vi "LaserSync_VI.vi"() -> ()   [LabVIEW 2015]
uses:
  <vilib>/Platform/TimedLoop/XDataNode/timing_clust.ctl
  <vilib>/Platform/TimedLoop/XDataNode/nitl_modes.ctl
  <vilib>/Platform/TimedLoop/XDataNode/wakeup.ctl
  <vilib>/FPGAPlugInAG/myRIO-1950/niLvFpga_Open_myRIO-1950.vi
  <vilib>/rvi/interface/common/dynamic/niFpgaDynamicAddResources.vi
  <vilib>/Utility/error.llb/Error Cluster From Error Code.vi
  <vilib>/rvi/errors/niLvFpgaAdjustHostInterfaceError.vi
  <vilib>/RVI Host/nirviSupport.llb/nirviErrorClusterFromErrorCode.vi
  <vilib>/Analysis/3filter.llb/Butterworth Filter (DBL).vi
  <vilib>/FPGAPlugInAG/Dynamic/niLvFpga_Close_Dynamic.vi
  <vilib>/Analysis/Matrix/Numeric/Conversions/Array To Matrix - RA.vi
  <vilib>/Platform/TimedLoop/XDataNode/XDataNode.xnode
  <vilib>/rvi/interface/nirviOpenFPGA/nirviOpenFPGA.xnode
  FPGA Bitfiles/Flylaserbox_FPGATarget_FPGAsingleloop_H8b3XToqd60.lvbitx
  FPGA_single_loop.vi
  <vilib>/rvi/interface/nirviReadWriteControl/nirviReadWriteControl.xnode
  <vilib>/rvi/interface/nirviMethod/nirviMethod.xnode
  <vilib>/rvi/interface/nirviCloseFPGA/nirviCloseFPGA.xnode
  <vilib>/Platform/TimedLoop/XDataNode/XDNodeRunTimeDep.lvlib
  <vilib>/rvi/interface/Simulation/niFpgaSimulationCallBeginRW.vi
  <vilib>/rvi/interface/nirviMethod/StockFPGA_InlinedMethodWaitForSingleIRQ.vi
  <vilib>/FPGAPlugInAG/Dynamic/niLvFpga_WaitOnIrq_Dynamic.vi
  <vilib>/FPGAPlugInAG/Dynamic/niLvFpga_ReadFifo_Dynamic.vi
  <vilib>/rvi/errors/niLvFpgaMergeErrorWithErrorCode.vi
  <vilib>/FPGAPlugInAG/Dynamic/niLvFpga_AcknowledgeIrq_Dynamic.vi
  <vilib>/Analysis/NI_AALBase.lvlib
  <vilib>/Analysis/Matrix/NI_Matrix.lvlib
  NiFpgaLv.dll
panel:
  in  "Laser On? All lasers":bool
  in  "Laser J8":u16=2855
  in  "Laser J5":u16=749
  in  "Laser J4":u16=766
  in  "Laser J1":u16=3000
  out "Loop count of LED":i32=6674
  in  "Producer Loop Stop-2":bool
  in  "Producer Loop Stop":bool
  out "Consumer Loop Time":u32=20
  out "Host VI loop count":i32=33366
  out "Noise check":dbl[](graph)
  out "Fly real-time location":dbl(graph)=245.7942691305756
  in  "Choose which setup to look at":dbl=2.0
  out "Display Raw Data":dbl[](graph)=[329.0, 351.0, 375.0, 381.0, 409.0, 416.0, 442.0, 448.0, 474.0, 481.0, 503.0, 511.0, 538.0, 543.0, 569.0, 571.0, 596.0, 603.0, 622.0, 627.0, 644.0, 647.0, 671.0, 666.0, 687.0, 687.0, 703.0, 701.0, 719.0, 713.0, 728.0, 726.0, 740.0, 733.0, 743.0, 736.0, 749.0, 742.0, 754.0, 743.0, 751.0, 742.0, 752.0, 741.0, 755.0, 747.0, 758.0, 752.0, 763.0, 754.0, 764.0, 757.0, 772.0, 762.0, 774.0, 766.0, 779.0, 769.0, 780.0, 770.0, 782.0, 770.0, 779.0, 769.0, 781.0, 773.0, 788.0, 777.0, 788.0, 780.0, 794.0, 785.0, 799.0, 792.0, 806.0, 801.0, 813.0, 808.0, 821.0, 814.0, 828.0, 821.0, 833.0, 826.0, 838.0, 830.0, 842.0, 830.0, 840.0, 834.0, 848.0, 838.0, 849.0, 837.0, 849.0, 840.0, 854.0, 842.0, 853.0, 848.0, 861.0, 849.0, 860.0, 854.0, 868.0, 855.0, 867.0, 859.0, 872.0, 863.0, 873.0, 865.0, 881.0, 871.0, 883.0, 874.0, 883.0, 877.0, 889.0, 880.0, 892.0, 879.0, 895.0, 887.0, 897.0, 885.0, 891.0, 881.0, 883.0, 894.0, 900.0, 897.0, 908.0, 907.0, 915.0, 912.0, 923.0, 921.0, 927.0, 926.0, 936.0, 934.0, 938.0, 937.0, 943.0, 936.0, 945.0, 941.0, 949.0, 943.0, 954.0, 951.0, 963.0, 960.0, 969.0, 968.0, 977.0, 974.0, 983.0, 981.0, 989.0, 986.0, 998.0, 991.0, 999.0, 995.0, 1002.0, 1002.0, 1004.0, 1002.0, 1006.0, 1002.0, 1014.0, 1007.0, 1016.0, 1013.0, 1020.0, 1013.0, 1022.0, 1015.0, 1019.0, 1016.0, 1021.0, 1018.0, 1022.0, 1015.0, 1021.0, 1012.0, 1019.0, 1013.0, 1015.0, 1014.0, 1018.0, 1009.0, 1019.0, 1014.0, 1019.0, 1015.0, 1020.0, 1016.0, 1024.0, 1012.0, 1020.0, 1013.0, 1017.0, 1015.0, 1025.0, 1020.0, 1029.0, 1021.0, 1027.0, 1023.0, 1028.0, 1018.0, 1025.0, 1021.0, 1026.0, 1017.0, 1019.0, 1013.0, 1016.0, 1004.0, 1007.0, 1006.0, 1007.0, 1000.0, 1001.0, 989.0, 994.0, 985.0, 989.0, 986.0, 988.0, 983.0, 987.0, 979.0, 983.0, 978.0, 984.0, 976.0, 984.0, 975.0, 983.0, 978.0, 983.0, 978.0, 986.0, 981.0, 984.0, 970.0, 978.0, 975.0, 981.0, 973.0, 968.0, 951.0, 999.0, 1012.0, 1013.0, 1012.0, 1009.0, 1010.0, 1012.0, 1017.0, 1016.0, 1019.0, 1021.0, 1028.0, 1030.0, 1035.0, 1037.0, 1043.0, 1047.0, 1052.0, 1054.0, 1061.0, 1064.0, 1069.0, 1074.0, 1080.0, 1082.0, 1087.0, 1089.0, 1091.0, 1095.0, 1099.0, 1096.0, 1098.0, 1099.0, 1103.0, 1106.0, 1110.0, 1112.0, 1115.0, 1119.0, 1124.0, 1123.0, 1127.0, 1127.0, 1130.0, 1132.0, 1134.0, 1134.0, 1137.0, 1134.0, 1137.0, 1139.0, 1139.0, 1139.0, 1139.0, 1138.0, 1142.0, 1141.0, 1139.0, 1139.0, 1139.0, 1135.0, 1135.0, 1133.0, 1138.0, 1137.0, 1137.0, 1136.0, 1135.0, 1131.0, 1133.0, 1131.0, 1132.0, 1129.0, 1129.0, 1127.0, 1126.0, 1119.0, 1120.0, 1120.0, 1119.0, 1115.0, 1114.0, 1111.0, 1109.0, 1107.0, 1106.0, 1104.0, 1102.0, 1102.0, 1102.0, 1101.0, 1098.0, 1097.0, 1097.0, 1095.0, 1103.0, 1095.0, 1097.0, 1095.0, 1099.0, 1099.0, 1101.0, 1099.0, 1105.0, 1104.0, 1105.0, 1110.0, 1112.0, 1112.0, 1114.0, 1116.0, 1114.0, 1114.0, 1113.0, 1116.0, 1118.0, 1117.0, 1119.0, 1117.0, 1121.0, 1122.0, 1123.0, 1123.0, 1125.0, 1122.0, 1127.0, 1130.0, 1127.0, 1118.0, 1129.0, 1126.0, 1125.0, 1114.0, 1114.0, 1107.0, 1109.0, 1101.0, 1105.0, 1101.0, 1103.0, 1097.0, 1103.0, 1097.0, 1105.0, 1098.0, 1099.0, 1096.0, 1101.0, 1099.0, 1103.0, 1101.0, 1105.0, 1099.0, 1104.0, 1101.0, 1106.0, 1098.0, 1101.0, 1096.0, 1098.0, 1091.0, 1096.0, 1093.0, 1097.0, 1094.0, 1098.0, 1093.0, 1099.0, 1093.0, 1099.0, 1096.0, 1102.0, 1102.0, 1108.0, 1107.0, 1113.0, 1110.0, 1114.0, 1114.0, 1120.0, 1116.0, 1122.0, 1120.0, 1128.0, 1125.0, 1131.0, 1130.0, 1136.0, 1131.0, 1135.0, 1133.0, 1140.0, 1137.0, 1143.0, 1139.0, 1141.0, 1138.0, 1139.0, 1137.0, 1145.0, 1142.0, 1144.0, 1138.0, 1149.0, 1148.0, 1153.0, 1147.0, 1150.0, 1145.0, 1149.0, 1144.0, 1147.0, 1140.0, 1144.0, 1139.0, 1144.0, 1137.0, 1142.0, 1139.0, 1144.0, 1139.0, 1142.0, 1137.0, 1142.0, 1138.0, 1144.0, 1141.0, 1144.0, 1143.0, 1150.0, 1147.0, 1156.0, 1154.0, 1157.0, 1157.0, 1161.0, 1157.0, 1162.0, 1160.0, 1166.0, 1160.0, 1168.0, 1163.0, 1171.0, 1166.0, 1170.0, 1165.0, 1171.0, 1167.0, 1170.0, 1165.0, 1169.0, 1165.0, 1172.0, 1170.0, 1185.0, 1094.0, 1101.0, 1108.0, 1099.0, 1106.0, 1104.0, 1101.0, 1100.0, 1103.0, 1099.0, 1099.0, 1094.0, 1098.0, 1089.0, 1093.0, 1086.0, 1088.0, 1081.0, 1083.0, 1078.0, 1082.0, 1074.0, 1074.0, 1069.0, 1073.0, 1066.0, 1065.0, 1060.0, 1065.0, 1058.0, 1060.0, 1055.0, 1053.0, 1053.0, 1053.0, 1047.0, 1048.0, 1043.0, 1051.0, 1045.0, 1047.0, 1042.0, 1045.0, 1038.0, 1043.0, 1038.0, 1040.0, 1038.0, 1044.0, 1041.0, 1043.0, 1037.0, 1042.0, 1037.0, 1036.0, 1035.0, 1040.0, 1033.0, 1039.0, 1033.0, 1036.0, 1035.0, 1036.0, 1032.0, 1032.0, 1032.0, 1035.0, 1028.0, 1036.0, 1034.0, 1037.0, 1032.0, 1034.0, 1031.0, 1033.0, 1030.0, 1034.0, 1026.0, 1028.0, 1026.0, 1030.0, 1022.0, 1028.0, 1021.0, 1023.0, 1020.0, 1019.0, 1014.0, 1012.0, 1009.0, 1010.0, 1004.0, 1008.0, 1002.0, 1003.0, 995.0, 997.0, 987.0, 991.0, 989.0, 987.0, 978.0, 978.0, 974.0, 978.0, 970.0, 973.0, 964.0, 964.0, 958.0, 961.0, 956.0, 954.0, 948.0, 950.0, 946.0, 945.0, 939.0, 938.0, 934.0, 935.0, 930.0, 928.0, 921.0, 923.0, 911.0, 905.0, 898.0, 899.0, 917.0, 903.0, 915.0, 901.0, 913.0, 899.0, 914.0, 897.0, 908.0, 894.0, 906.0, 889.0, 903.0, 887.0, 900.0, 884.0, 899.0, 880.0, 892.0, 877.0, 886.0, 875.0, 887.0, 870.0, 883.0, 868.0, 878.0, 862.0, 875.0, 861.0, 873.0, 857.0, 867.0, 850.0, 864.0, 848.0, 859.0, 844.0, 853.0, 837.0, 847.0, 829.0, 840.0, 822.0, 829.0, 810.0, 822.0, 805.0, 814.0, 802.0, 814.0, 801.0, 814.0, 799.0, 811.0, 797.0, 809.0, 793.0, 803.0, 790.0, 798.0, 788.0, 798.0, 783.0, 794.0, 780.0, 787.0, 776.0, 788.0, 772.0, 781.0, 772.0, 780.0, 767.0, 780.0, 768.0, 771.0, 760.0, 770.0, 751.0, 763.0, 749.0, 761.0, 743.0, 741.0, 709.0, 722.0, 730.0, 737.0, 728.0, 737.0, 724.0, 732.0, 719.0, 723.0, 712.0, 717.0, 701.0, 704.0, 690.0, 695.0, 678.0, 682.0, 664.0, 666.0, 647.0, 645.0, 623.0, 626.0, 606.0, 603.0, 581.0, 576.0, 554.0, 551.0, 529.0, 520.0, 499.0, 490.0, 471.0, 462.0, 443.0, 433.0, 414.0, 405.0, 381.0, 374.0, 268.0, 323.0]
  in  "Fly presence? J8":bool=TRUE
  in  "Threshhold position filter J8":i32=25
  in  "Fly presence? J5":bool=TRUE
  in  "Threshhold position filter J5":i32=25
  in  "Fly presence? J4":bool=TRUE
  in  "Threshhold position filter J4":i32=25
  in  "Threshhold position filter J1":i32=25
  in  "Fly presence? J1":bool=TRUE
  in  "Threshold for noise filter J4":dbl=7.0
  in  "Threshold for noise filter J5":dbl=6.0
  in  "Threshold for noise filter J8":dbl=8.0
  in  "Threshold for noise filter J1":dbl=8.0
  in  "Consumer Loop Stop":bool
  out "Has timed loop ever been late?":bool
  out "Finished Late? [i-1]":bool
  in  "Sensor loop time":i64=20
  in  "Gender J4":string="M"
  in  "Date":string="2017June25"
  in  "Testname J4":string="A"
  in  "Gender J8":string="M"
  in  "Date":string="2017June25"
  in  "Fly J8":i32=4
  in  "Testname Code J8":string="A"
  in  "Fly J4":i32=2
  in  "Gender J5":string="M"
  in  "Date":string="2017June25"
  in  "Fly J5":i32=3
  in  "Testname Code J5":string="A"
  in  "Gender J1":string="F"
  in  "Date":string="2017June25"
  in  "Fly J1":i32=1
  in  "Testname J1":string="A"
  in  "FPGA Stop":bool
  in  "LED switch-2 J8":bool=TRUE
  in  "LED switch-1 J8":bool=TRUE
  in  "LED switch-2 J5":bool=TRUE
  in  "LED switch-1 J5":bool=TRUE
  in  "LED switch-2 J4":bool=TRUE
  in  "LED switch-1 J4":bool=TRUE
  in  "LED switch-2 J1":bool=TRUE
  in  "LED switch-1 J1":bool=TRUE
  in  "LED intensity J8":u32=1000
  in  "LED intensity J5":u32=1000
  in  "LED intensity J4":u32=2500
  in  "LED intensity J1":u32=1000
  out "Frame Count":i16=6056
  out "Host loop time":u32=13
  in  "FIFO Timeout setting (ms)":i32=5000
  out "Elements Remaining Real":u32
  out "Elements Remaining":u32=3080
  out "IRQ(s) Asserted":i32
  out "Sensor Loop Time (FPGA)":u32=11
  out "LED loop time":u32=4000
  out "Iteration Duration":dbl=4.0 format="%#_6f"
  # "0: None\n1: J1\n2: J4\n3: J5\n4: J8"
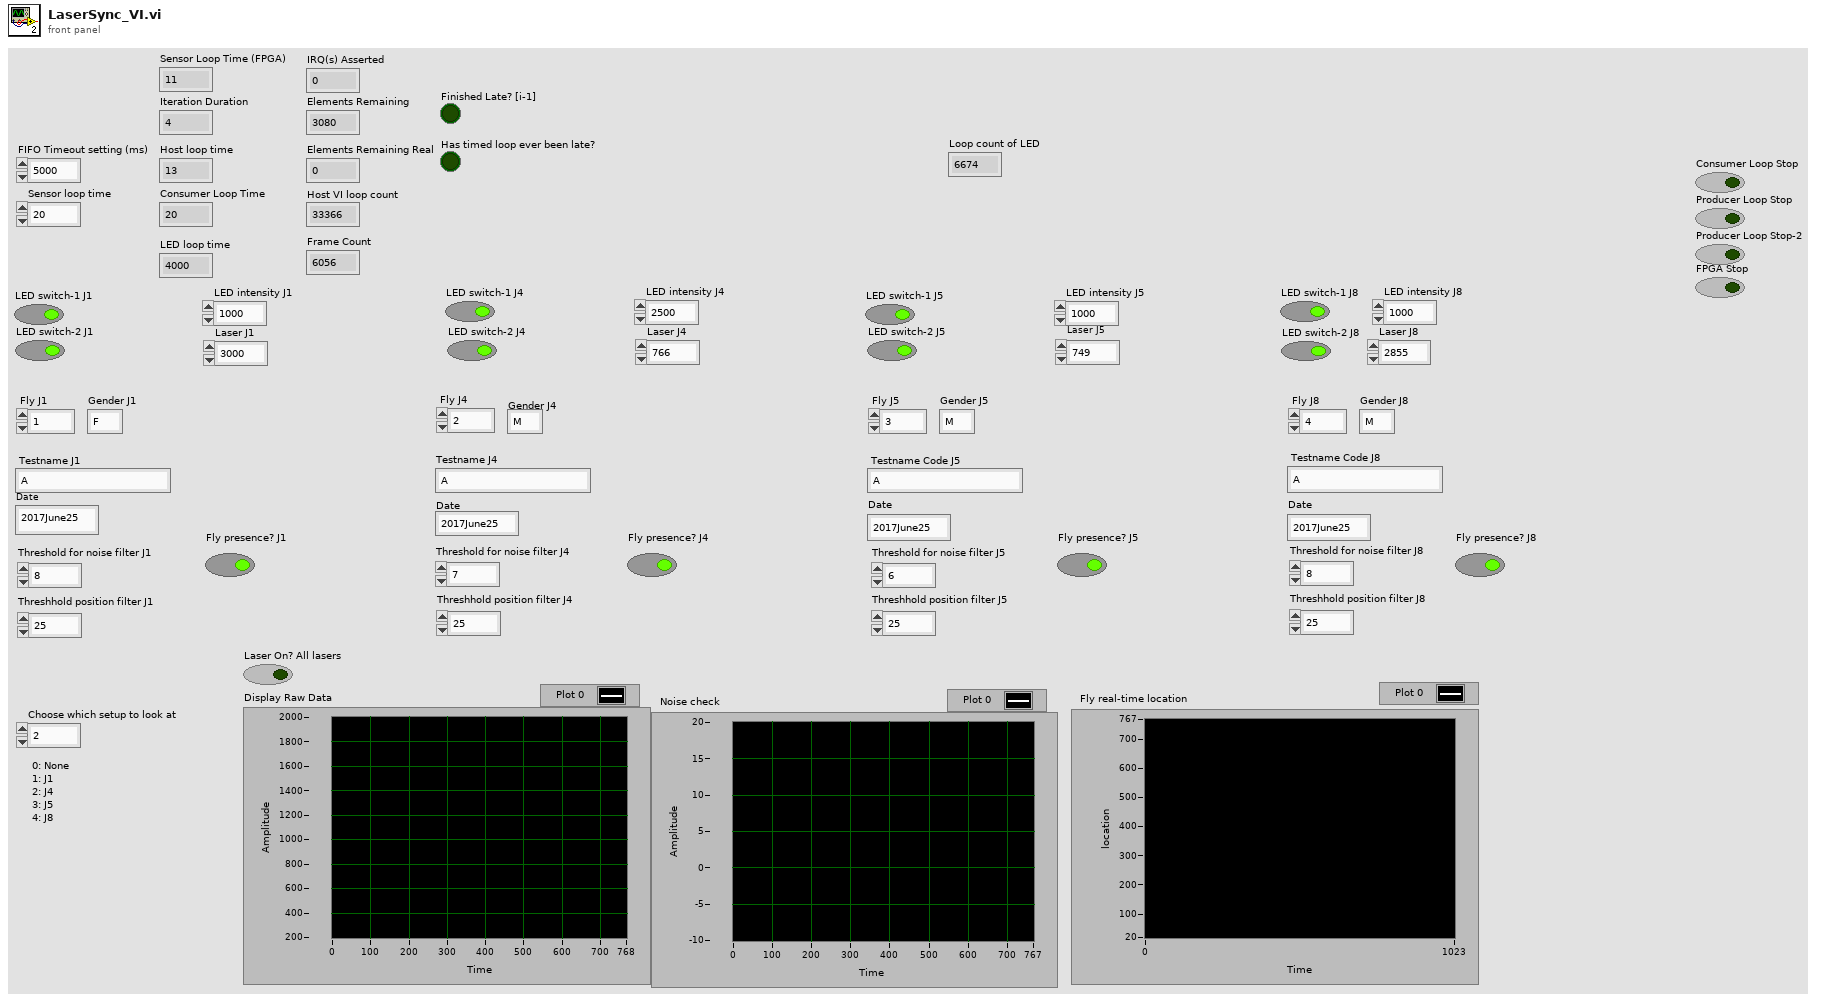
[diagram p1: front panel]
types:
  T1 = enum16{"open", "open or create", "create or replace", "create", "open (read-only)"}
  T2 = typedef "XDNodeRunTimeDep.lvlib/timing_clust.ctl" = cluster{"Expected End [f-1]":u64, "Actual End [f-1]":u64, "Finished Late? [f-1]":bool, "Expected End [i-1]":u64, "Actual End [i-1]":u64, "Finished Late? [i-1]":bool, "Expected Start [i]":u64, "Actual Start [i]":u64, "Expected Start [f]":u64, "Actual Start [f]":u64, "Source Name":string, "Structure Name":string, "Period":i64, "Deadline":i64, "Offset":i64, "Start":i64, "Priority":i32, "Timeout":i32, "Mode":T3, "Wakeup Reason":T4, "Error":errorcluster, "Source Type":string, "Secondary Source Type":string, "Global End Time":u64, "Global Start Time":u64, "Frame Duration":u64, "Iteration Duration":u64, "Assigned CPU":i32, "I/O Scan Engine Mode":u32}
  T3 = typedef "XDNodeRunTimeDep.lvlib/nitl_modes.ctl" = enum32{"No Change", "Process missed periods, maintain original phase", "Discard missed periods, maintain original phase", "Process missed periods, ignore original phase", "Discard missed periods, ignore original phase"}
  T4 = typedef "XDNodeRunTimeDep.lvlib/wakeup.ctl" = enum32{"Normal", "Aborted", "Asynchronous wakeup", "Timing source error", "Timed loop error", "Timeout"}
  T5 = typedef "NI_Matrix.lvlib/RealMatrix.ctl" = dbl[][]
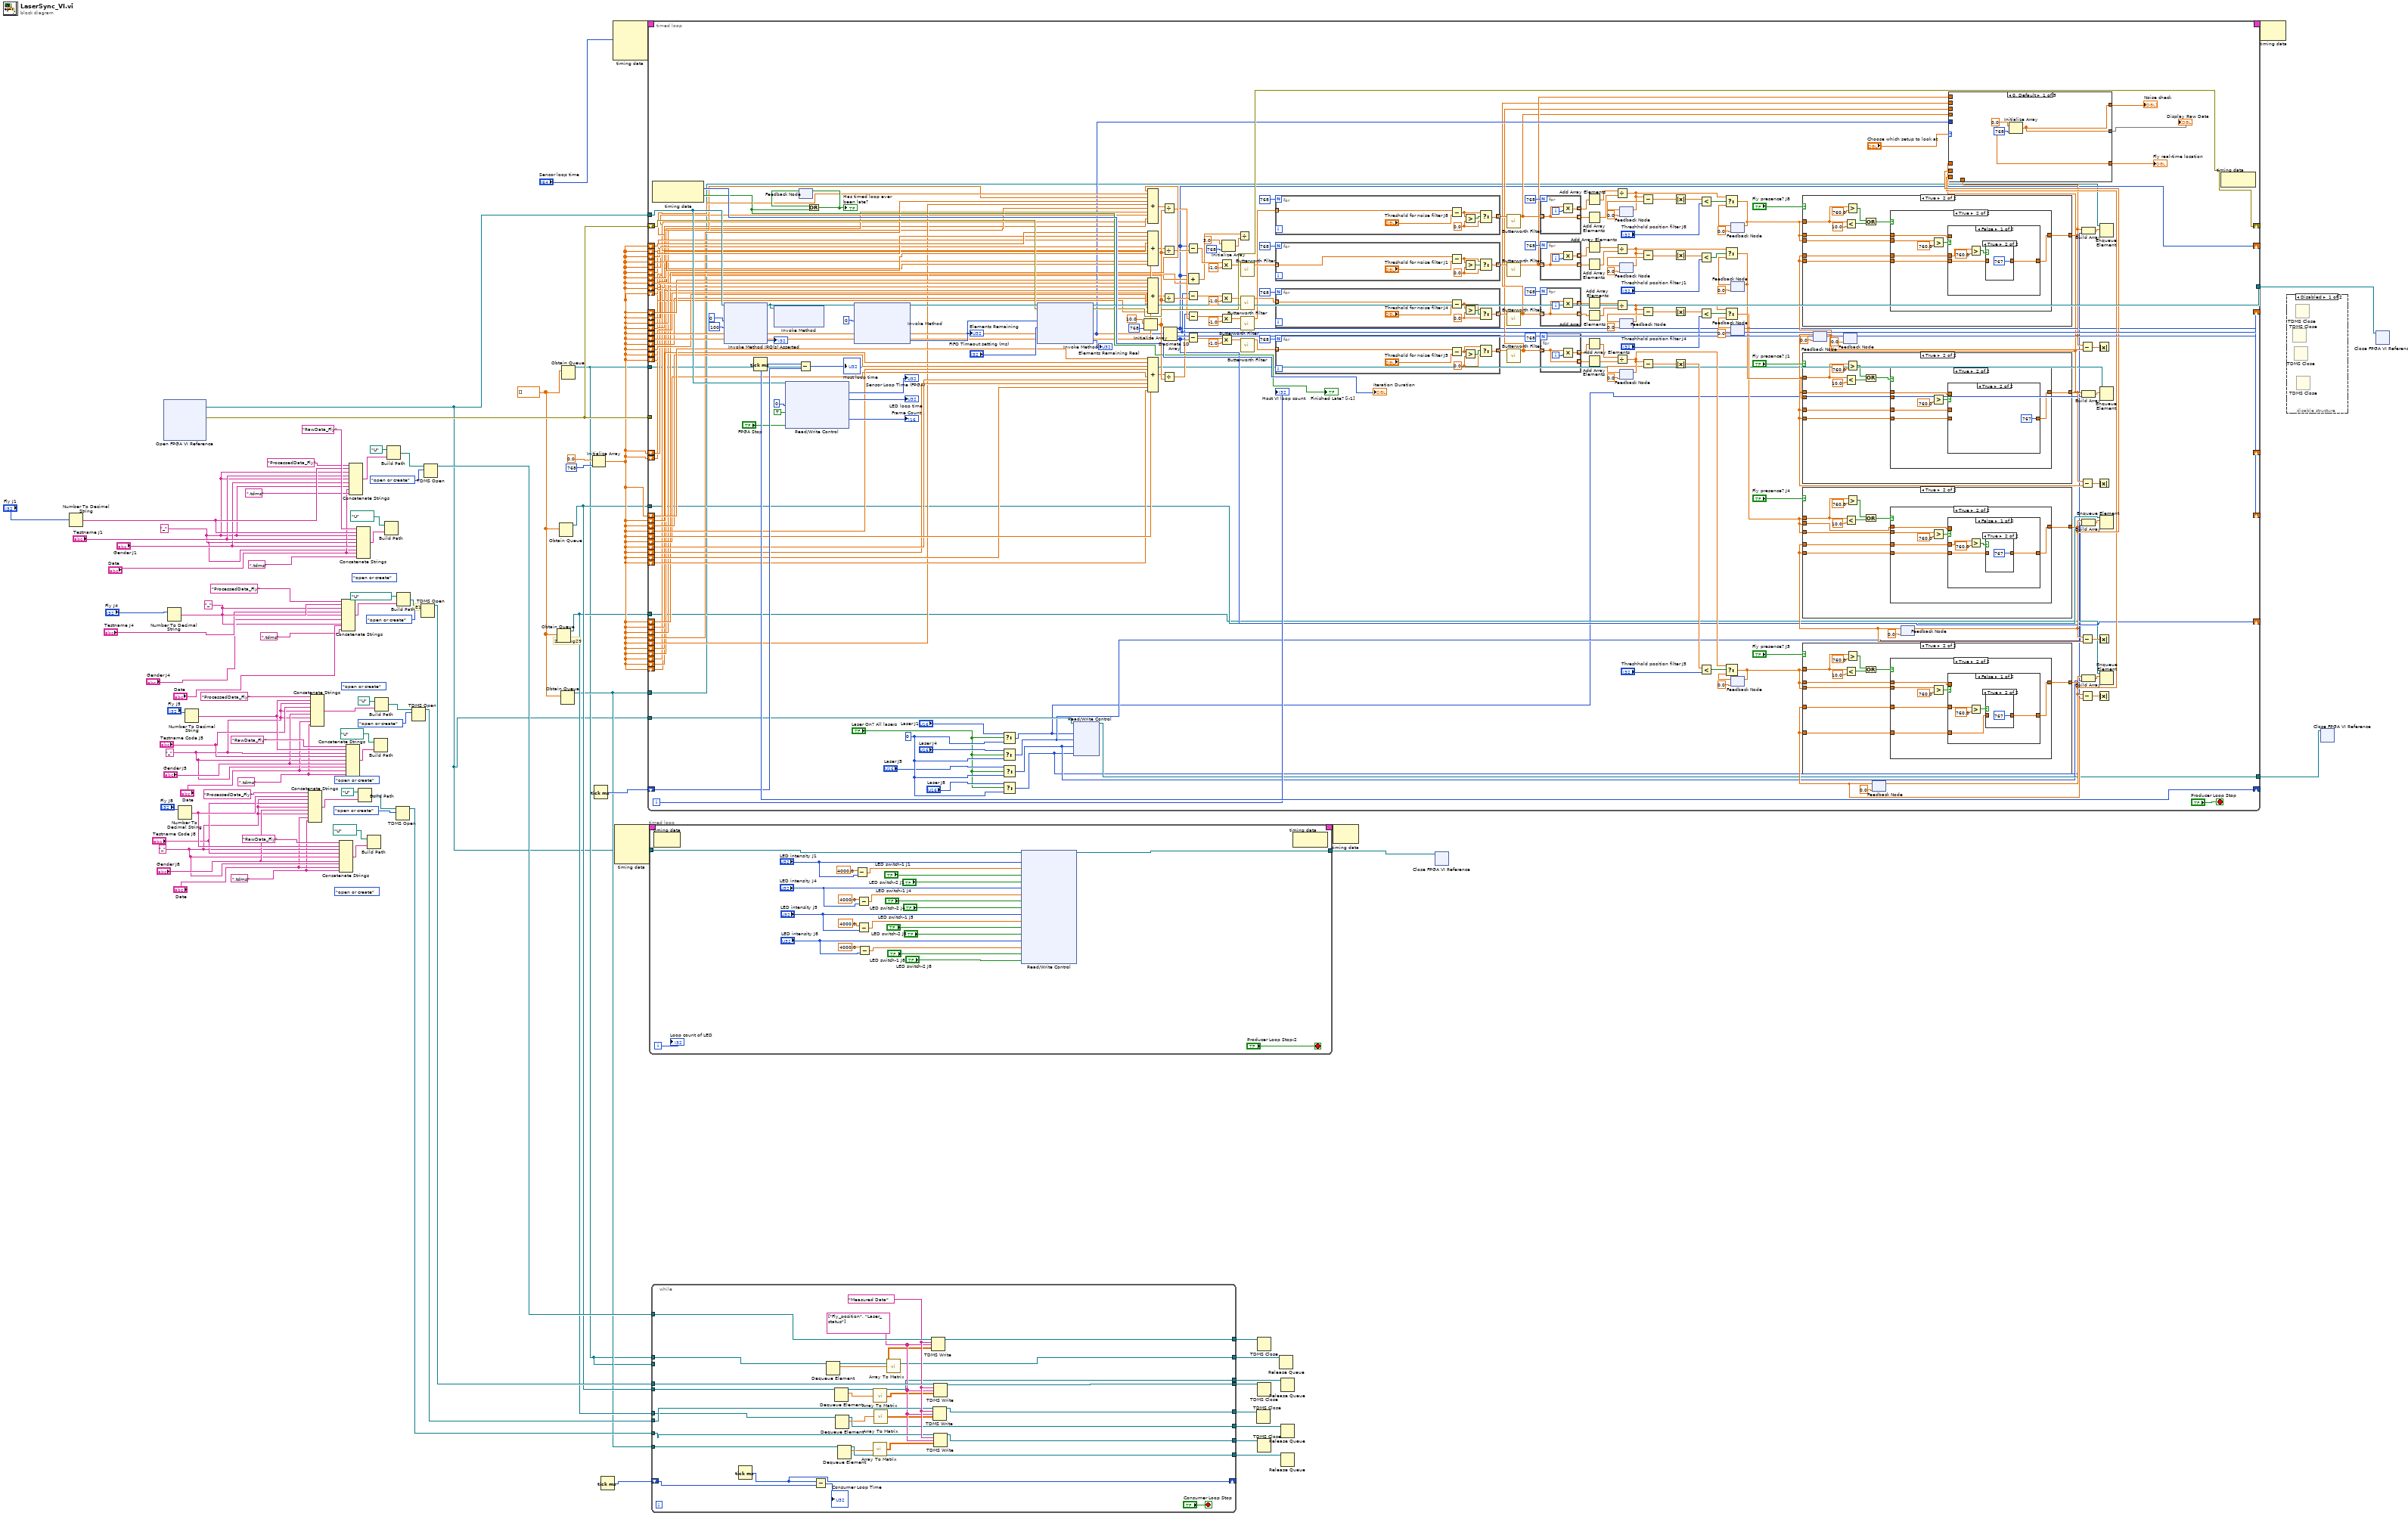
[diagram p0: block diagram]
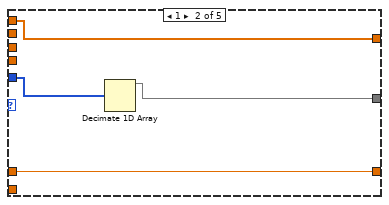
[diagram p3: hidden frame]
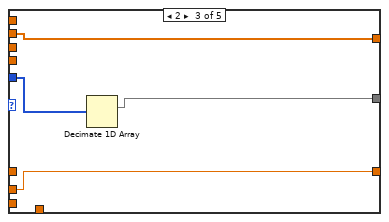
[diagram p4: hidden frame]
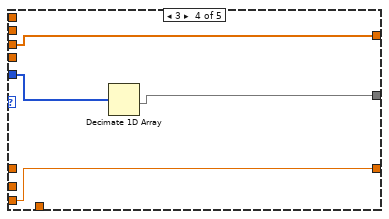
[diagram p5: hidden frame]
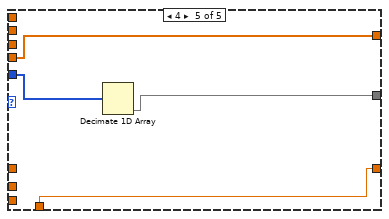
[diagram p6: hidden frame]
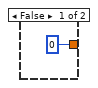
[diagram p7: hidden frame]
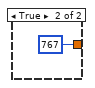
[diagram p10: hidden frame]
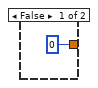
[diagram p11: hidden frame]
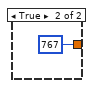
[diagram p14: hidden frame]
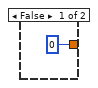
[diagram p15: hidden frame]
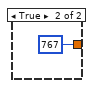
[diagram p18: hidden frame]
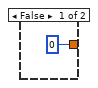
[diagram p19: hidden frame]
diagram:
  w8 = dbl[] [] ("appended array")
  w29 = "_" ("string")
  w27 = ".tdms" ("string")
  (unwired) T1."open or create" ("operation (0:open)")
  w39 = "_" ("string")
  w38 = ".tdms" ("string")
  (unwired) T1."open or create" ("operation (0:open)")
  w51 = "_" ("string")
  (unwired) T1."open or create" ("operation (0:open)")
  w60 = "_" ("string")
  (unwired) T1."open or create" ("operation (0:open)")
  # "2018Aug29"
  # "E1"
  n1 = Number To Decimal String(number="Fly J1") -> (decimal integer string=w65:string)  [unwired: 1 in]
  n2 = xnode "Open FPGA VI Reference"() -> ("FPGA VI Reference Out"=w2:refnum<k20>, "error out"=w22:errorcluster)  [unwired: 2 in]
  n3 = Number To Decimal String(number="Fly J4") -> (decimal integer string=w54:string)  [unwired: 1 in]
  n4 = Number To Decimal String(number="Fly J8") -> (decimal integer string=w32:string)  [unwired: 1 in]
  n5 = Number To Decimal String(number="Fly J5") -> (decimal integer string=w43:string)  [unwired: 1 in]
  n6 = Concatenate Strings("ProcessedData_Fly" ("string"), w32, w29, "Testname Code J8", w29, "Gender J8", w29, "Date", w27) -> (w23:string)
  n7 = Concatenate Strings("ProcessedData_Fly" ("string"), w43, w39, "Testname Code J5", w39, "Gender J5", w39, "Date", w38) -> (w34:string)
  n8 = Concatenate Strings("RawData_Fly" ("string"), w32, w29, "Testname Code J8", w29, "Gender J8", w29, "Date", w27) -> (w70:string)
  n9 = Concatenate Strings("ProcessedData_Fly" ("string"), w54, w51, "Testname J4", w51, "Gender J4", w51, "Date", ".tdms" ("string")) -> (w47:string)
  n10 = Concatenate Strings("RawData_Fly" ("string"), w43, w39, "Testname Code J5", w39, "Gender J5", w39, "Date", w38) -> (w75:string)
  n11 = Concatenate Strings("ProcessedData_Fly" ("string"), w65, w60, "Testname J1", w60, "Gender J1", w60, "Date", ".tdms" ("string")) -> (w57:string)
  n12 = Concatenate Strings("RawData_Fly" ("string"), w65, w60, "Testname J1", w60, "Gender J1", w60, "Date", ".tdms" ("string")) -> (w80:string)
  n13 = Build Path(base path=path "U:/", name or relative path=w23) -> (appended path=w25:path)
  n14 = Build Path(base path=path "U:/", name or relative path=w70) -> ()  [unwired: 1 out]
  n15 = Build Path(base path=path "U:/", name or relative path=w75) -> ()  [unwired: 1 out]
  n16 = Build Path(base path=path "U:/", name or relative path=w34) -> (appended path=w36:path)
  n17 = Build Path(base path=path "U:/", name or relative path=w80) -> ()  [unwired: 1 out]
  n18 = Build Path(base path=path "U:/", name or relative path=w57) -> (appended path=w58:path)
  n19 = TDMS Open(10:T1."open or create" ("operation (0:open)"), 11:w25) -> (3:w16:refnum<k34>)  [unwired: 5 in, 1 out]
  n20 = Build Path(base path=path "U:/", name or relative path=w47) -> (appended path=w45:path)
  n21 = TDMS Open(10:T1."open or create" ("operation (0:open)"), 11:w36) -> (3:w15:refnum<k34>)  [unwired: 5 in, 1 out]
  n22 = TDMS Open(10:T1."open or create" ("operation (0:open)"), 11:w45) -> (3:w14:refnum<k34>)  [unwired: 5 in, 1 out]
  n23 = TDMS Open(10:T1."open or create" ("operation (0:open)"), 11:w58) -> (3:w17:refnum<k34>)  [unwired: 5 in, 1 out]
  n24 = Obtain Queue(element data type=w8) -> (queue out=w7:refnum<queue>)  [unwired: 4 in, 2 out]
  n25 = Obtain Queue(element data type=w8) -> (queue out=w12:refnum<queue>)  [unwired: 4 in, 2 out]
  n26 = Obtain Queue(element data type=w8) -> (queue out=w6:refnum<queue>)  [unwired: 4 in, 2 out]
  n27 = Obtain Queue(element data type=w8) -> (queue out=w4:refnum<queue>)  [unwired: 4 in, 2 out]
  n28 = Initialize Array(0.0 ("element"), 768 ("dimension size")) -> (w13:dbl[])
  n29 = Tick Count (ms)() -> (millisecond timer value=w88:u32)
  n30 = Tick Count (ms)() -> (millisecond timer value=w3:u32)
  n31 = node-c288("Sensor loop time") -> (w90:T2)  [unwired: 3 in]
  n32 = node-c288() -> (w85:T2)  [unwired: 4 in]
  n33 = timed-loop {
    tunnel: w2 -> [w296]
    shift-right: [w311] -> _
    shift-left: w88 -> [w310]
    timing: w90 -> [_]
    timing-out: [_] -> w89
    tunnel: [w297] -> w87
    shift-right: [w235] -> _
    shift-left: w13 -> [w276]
    shift-left: w13 -> [w275]
    shift-left: w13 -> [w274]
    shift-left: w13 -> [w273]
    shift-left: w13 -> [w272]
    shift-left: w13 -> [w271]
    shift-left: w13 -> [w270]
    shift-left: w13 -> [w269]
    shift-left: w13 -> [w268]
    shift-left: w13 -> [w267]
    shift-right: [w113] -> _
    shift-left: w13 -> [w256]
    shift-left: w13 -> [w255]
    shift-left: w13 -> [w254]
    shift-left: w13 -> [w253]
    shift-left: w13 -> [w252]
    shift-left: w13 -> [w251]
    shift-left: w13 -> [w250]
    shift-left: w13 -> [w249]
    shift-left: w13 -> [w248]
    shift-left: w13 -> [w247]
    shift-right: [w234] -> _
    shift-left: w13 -> [w266]
    shift-left: w13 -> [w265]
    shift-left: w13 -> [w264]
    shift-left: w13 -> [w263]
    shift-left: w13 -> [w262]
    shift-left: w13 -> [w261]
    shift-left: w13 -> [w260]
    shift-left: w13 -> [w259]
    shift-left: w13 -> [w258]
    shift-left: w13 -> [w257]
    shift-right: [w114] -> _
    shift-left: w13 -> [w286]
    shift-left: w13 -> [w285]
    shift-left: w13 -> [w284]
    shift-left: w13 -> [w283]
    shift-left: w13 -> [w282]
    shift-left: w13 -> [w281]
    shift-left: w13 -> [w280]
    shift-left: w13 -> [w279]
    shift-left: w13 -> [w278]
    shift-left: w13 -> [w277]
    tunnel: w22 -> [_]
    shift-right: [w288] -> _
    shift-left: w22 -> [w287]
    shift-right: [w114] -> _
    shift-left: w13 -> [w120]
    shift-left: w13 -> [w119]
    tunnel: w4 -> [w104]
    tunnel: w12 -> [w110]
    tunnel: w7 -> [w107]
    tunnel: w6 -> [w106]
    tunnel: w2 -> [w96]
    tunnel: [w95] -> w1
    i -> [w121]
    stop <- "Producer Loop Stop" stop-if-true
    w101 = 0
    n34 = node-c288() -> (→"Iteration Duration":i64, w292:bool)  [unwired: 1 in]
    "Finished Late? [i-1]" <- w292
    n35 = xnode "Invoke Method"("FPGA VI Reference In"=w296, "IRQ Number(s)"=0, "Timeout (ms)"=100) -> ("FPGA VI Reference Out"=w290:refnum<k20>, "IRQ(s) Asserted"=→"IRQ(s) Asserted":i32)  [unwired: 1 in, 2 out]
    n36 = Tick Count (ms)() -> (millisecond timer value=w311:u32)
    n37 = xnode "Invoke Method"("FPGA VI Reference In"=w290) -> ()  [unwired: 2 in, 2 out]
    n38 = xnode "Read/Write Control"("FPGA VI Reference In"=w296, "IRQ Bit (0-31)"=u8 0 ("IRQ Bit (0-31) J1"), "Wait Until IRQ Cleared?"=TRUE ("Wait Until IRQ Cleared? J1"), "FPGA Stop"="FPGA Stop") -> ("Sensor Loop Time"=→"Sensor Loop Time (FPGA)":u32, "LED loop time"=→"LED loop time":u32, "Frame Count"=→"Frame Count":i16)  [unwired: 1 in, 2 out]
    n39 = feedback #1() -> (w294:bool)  [unwired: 1 in]
    n40 = Subtract(x=w311, y=w310) -> (x-y=→"Host loop time":u32)
    n41 = Or(x=w294, y=w292) -> (x .or. y?=w295:bool)
    "Has timed loop ever been late?" <- w295
    n42 = feedback-in #1(w295) -> ()
    n43 = xnode "Invoke Method"("FPGA VI Reference In"=w290, "Number of Elements"=u32 0) -> ("FPGA VI Reference Out"=w299:refnum<k20>, "Elements Remaining"=w298:u32)  [unwired: 2 in, 2 out]
    "Elements Remaining" <- w298
    n44 = Select(t="Laser J1", s="Laser On? All lasers", f=w101) -> (s? t:f=w93:i32)
    n45 = Select(t="Laser J4", s="Laser On? All lasers", f=w101) -> (s? t:f=w94:i32)
    n46 = Select(t="Laser J5", s="Laser On? All lasers", f=w101) -> (s? t:f=w92:i32)
    n47 = Select(t="Laser J8", s="Laser On? All lasers", f=w101) -> (s? t:f=w91:i32)
    n48 = xnode "Invoke Method"("FPGA VI Reference In"=w299, "error in"=w287, "Number of Elements"=w298, "Timeout (ms)"="FIFO Timeout setting (ms)") -> ("FPGA VI Reference Out"=w297:refnum<k20>, "error out"=w288:errorcluster, "Data"=w133:u16[], "Elements Remaining"=→"Elements Remaining Real":u32)
    n49 = xnode "Read/Write Control"("FPGA VI Reference In"=w96, "Laser J1"=w93, "Laser J4"=w94, "Laser J5"=w92, "Laser J8"=w91) -> ("FPGA VI Reference Out"=w95:refnum<k20>)  [unwired: 1 in, 1 out]
    n50 = Initialize Array(10.0 ("element"), 768 ("dimension size")) -> (w244:dbl[])
    n51 = Compound Arithmetic op=ADD(w256, w255, w254, w253, w252, w251, w250, w249, w248, w247) -> (w240:dbl[])
    n52 = Compound Arithmetic op=ADD(w286, w285, w284, w283, w282, w281, w280, w279, w278, w277) -> (w243:dbl[])
    n53 = Compound Arithmetic op=ADD(w276, w275, w274, w273, w272, w271, w270, w269, w268, w267) -> (w242:dbl[])
    n54 = Compound Arithmetic op=ADD(w266, w265, w264, w263, w262, w261, w260, w259, w258, w257) -> (w241:dbl[])
    n55 = Divide(x=w240, y=w244) -> (x/y=w236:dbl[])
    n56 = Divide(x=w243, y=w244) -> (x/y=w239:dbl[])
    n57 = Divide(x=w242, y=w244) -> (x/y=w238:dbl[])
    n58 = Divide(x=w241, y=w244) -> (x/y=w237:dbl[])
    n59 = Decimate 1D Array(w133) -> (w114:u16[], w235:u16[], w234:u16[], w113:u16[])
    n60 = Subtract(x=w114, y=w239) -> (x-y=w230:dbl[])
    n61 = Subtract(x=w235, y=w238) -> (x-y=w231:dbl[])
    n62 = Subtract(x=w113, y=w236) -> (x-y=w233:dbl[])
    n63 = Subtract(x=w234, y=w237) -> (x-y=w232:dbl[])
    n64 = Compound Arithmetic op=ADD(w114, w120, w119) -> (w116:dbl[])
    n65 = Multiply(x=w230, y=-1.0) -> (x*y=w225:dbl[])
    n66 = Multiply(x=w231, y=-1.0) -> (x*y=w224:dbl[])
    n67 = Multiply(x=w233, y=-1.0) -> (x*y=w222:dbl[])
    n68 = Multiply(x=w232, y=-1.0) -> (x*y=w223:dbl[])
    n69 = Initialize Array(3.0 ("element"), 768 ("dimension size")) -> (w115:dbl[])
    n70 = Divide(x=w116, y=w115) -> ()  [unwired: 1 out]
    n71 = call-poly <vilib>:"Butterworth Filter.vi"("X"=w225) -> ("Filtered X"=w221:dbl[])  [unwired: 7 in, 1 out]
    n72 = call-poly <vilib>:"Butterworth Filter.vi"("X"=w224) -> ("Filtered X"=w218:dbl[])  [unwired: 7 in, 1 out]
    n73 = call-poly <vilib>:"Butterworth Filter.vi"("X"=w222) -> ("Filtered X"=w220:dbl[])  [unwired: 7 in, 1 out]
    n74 = call-poly <vilib>:"Butterworth Filter.vi"("X"=w223) -> ("Filtered X"=w219:dbl[])  [unwired: 7 in, 1 out]
    n75 = for {
      N: 768 -> [_]
      tunnel: w220 -> [w473] mode=indexing
      tunnel: [w469] -> w210 mode=indexing
      w470 = 0.0 ("y")
      n76 = Subtract(x=w473, y="Threshold for noise filter J8") -> (x-y=w471:dbl)
      n77 = Greater?(x=w471, y=w470) -> (0:w472:bool)
      n78 = Select(t=w471, s=w472, f=w470) -> (s? t:f=w469:dbl)
    }
    n79 = for {
      N: 768 -> [_]
      tunnel: w221 -> [w479] mode=indexing
      tunnel: [w475] -> w213 mode=indexing
      w476 = 0.0 ("y")
      n80 = Subtract(x=w479, y="Threshold for noise filter J1") -> (x-y=w477:dbl)
      n81 = Greater?(x=w477, y=w476) -> (0:w478:bool)
      n82 = Select(t=w477, s=w478, f=w476) -> (s? t:f=w475:dbl)
    }
    n83 = for {
      N: 768 -> [_]
      tunnel: w218 -> [w467] mode=indexing
      tunnel: [w463] -> w212 mode=indexing
      w464 = 0.0 ("y")
      n84 = Subtract(x=w467, y="Threshold for noise filter J4") -> (x-y=w465:dbl)
      n85 = Greater?(x=w465, y=w464) -> (0:w466:bool)
      n86 = Select(t=w465, s=w466, f=w464) -> (s? t:f=w463:dbl)
    }
    n87 = for {
      N: 768 -> [_]
      tunnel: w219 -> [w461] mode=indexing
      tunnel: [w457] -> w211 mode=indexing
      w458 = 0.0 ("y")
      n88 = Subtract(x=w461, y="Threshold for noise filter J5") -> (x-y=w459:dbl)
      n89 = Greater?(x=w459, y=w458) -> (0:w460:bool)
      n90 = Select(t=w459, s=w460, f=w458) -> (s? t:f=w457:dbl)
    }
    n91 = call-poly <vilib>:"Butterworth Filter.vi"("X"=w210) -> ("Filtered X"=w122:dbl[])  [unwired: 7 in, 1 out]
    n92 = call-poly <vilib>:"Butterworth Filter.vi"("X"=w213) -> ("Filtered X"=w125:dbl[])  [unwired: 7 in, 1 out]
    n93 = call-poly <vilib>:"Butterworth Filter.vi"("X"=w212) -> ("Filtered X"=w124:dbl[])  [unwired: 7 in, 1 out]
    n94 = call-poly <vilib>:"Butterworth Filter.vi"("X"=w211) -> ("Filtered X"=w123:dbl[])  [unwired: 7 in, 1 out]
    n95 = for {
      N: 768 -> [_]
      tunnel: w122 -> [w453] mode=indexing
      tunnel: [w454] -> w199 mode=indexing
      tunnel: [w453] -> w198 mode=indexing
      i -> [w455]
      n96 = Multiply(x=w453, y=w455) -> (x*y=w454:dbl)
    }
    n97 = for {
      N: 768 -> [_]
      tunnel: w125 -> [w450] mode=indexing
      tunnel: [w451] -> w205 mode=indexing
      tunnel: [w450] -> w204 mode=indexing
      i -> [w452]
      n98 = Multiply(x=w450, y=w452) -> (x*y=w451:dbl)
    }
    n99 = for {
      N: 768 -> [_]
      tunnel: w124 -> [w447] mode=indexing
      tunnel: [w448] -> w203 mode=indexing
      tunnel: [w447] -> w202 mode=indexing
      i -> [w449]
      n100 = Multiply(x=w447, y=w449) -> (x*y=w448:dbl)
    }
    n101 = for {
      N: 768 -> [_]
      tunnel: w123 -> [w444] mode=indexing
      tunnel: [w445] -> w201 mode=indexing
      tunnel: [w444] -> w200 mode=indexing
      i -> [w446]
      n102 = Multiply(x=w444, y=w446) -> (x*y=w445:dbl)
    }
    n103 = Add Array Elements(numeric array=w199) -> (sum=w191:dbl)
    n104 = Add Array Elements(numeric array=w198) -> (sum=w190:dbl)
    n105 = Add Array Elements(numeric array=w205) -> (sum=w197:dbl)
    n106 = Add Array Elements(numeric array=w204) -> (sum=w196:dbl)
    n107 = Add Array Elements(numeric array=w203) -> (sum=w195:dbl)
    n108 = Add Array Elements(numeric array=w202) -> (sum=w194:dbl)
    n109 = Add Array Elements(numeric array=w201) -> (sum=w193:dbl)
    n110 = Add Array Elements(numeric array=w200) -> (sum=w192:dbl)
    n111 = Divide(x=w191, y=w190) -> (x/y=w139:dbl)
    n112 = Divide(x=w197, y=w196) -> (x/y=w181:dbl)
    n113 = Divide(x=w195, y=w194) -> (x/y=w168:dbl)
    n114 = Divide(x=w193, y=w192) -> (x/y=w154:dbl)
    n115 = feedback #2(0.0) -> (w144:dbl)
    n116 = feedback-in #2(w139) -> ()
    n117 = feedback #3(0.0) -> (w183:dbl)
    n118 = feedback-in #3(w181) -> ()
    n119 = feedback #4(0.0) -> (w169:dbl)
    n120 = feedback-in #4(w168) -> ()
    n121 = feedback #5(0.0) -> (w153:dbl)
    n122 = feedback-in #5(w154) -> ()
    n123 = Subtract(x=w139, y=w144) -> (x-y=w147:dbl)
    n124 = Subtract(x=w181, y=w183) -> (x-y=w189:dbl)
    n125 = Subtract(x=w168, y=w169) -> (x-y=w176:dbl)
    n126 = Subtract(x=w154, y=w153) -> (x-y=w161:dbl)
    n127 = Absolute Value(x=w147) -> (abs(x)=w146:dbl)
    n128 = Absolute Value(x=w189) -> (abs(x)=w188:dbl)
    n129 = Absolute Value(x=w176) -> (abs(x)=w175:dbl)
    n130 = Absolute Value(x=w161) -> (abs(x)=w160:dbl)
    n131 = Less?(x=w146, y="Threshhold position filter J8") -> (x < y?=w145:bool)
    n132 = Less?(x=w188, y="Threshhold position filter J1") -> (x < y?=w186:bool)
    n133 = Less?(x=w175, y="Threshhold position filter J4") -> (x < y?=w173:bool)
    n134 = Less?(x=w160, y="Threshhold position filter J5") -> (x < y?=w156:bool)
    n135 = feedback #6(0.0) -> (w141:dbl)
    n136 = Select(t=w139, s=w145, f=w141) -> (s? t:f=w138:dbl)
    n137 = feedback-in #6(w138) -> ()
    n138 = feedback #7(0.0) -> (w185:dbl)
    n139 = Select(t=w181, s=w186, f=w185) -> (s? t:f=w180:dbl)
    n140 = feedback-in #7(w180) -> ()
    n141 = feedback #8(0.0) -> (w172:dbl)
    n142 = Select(t=w168, s=w173, f=w172) -> (s? t:f=w166:dbl)
    n143 = feedback-in #8(w166) -> ()
    n144 = feedback #9(0.0) -> (w157:dbl)
    n145 = Select(t=w154, s=w156, f=w157) -> (s? t:f=w151:dbl)
    n146 = feedback-in #9(w151) -> ()
    n147 = feedback #10(0.0) -> (w162:dbl)
    n148 = case shown="True" "Fly presence? J1" {
      tunnel: w180 -> [_ w427]
      tunnel: [0 w426] -> w112
      tunnel: w180 -> [_ w420]
      tunnel: w180 -> [_ w419]
      tunnel: w162 -> [_ w418]
      tunnel: w162 -> [_ w417]
      frame False {
      }
      frame True {
        n149 = Less?(x=w420, y=10.0) -> (x < y?=w423:bool)
        n150 = Greater?(x=w420, y=760.0) -> (0:w421:bool)
        n151 = Or(x=w421, y=w423) -> (x .or. y?=w425:bool)
        n152 = case shown="True" w425 {
          tunnel: w427 -> [w428 w434]
          tunnel: [w428 w435] -> w426
          tunnel: w419 -> [_ w429]
          tunnel: w418 -> [_ w432]
          tunnel: w417 -> [_ w430]
          frame False {
          }
          frame True {
            n153 = Greater?(x=w429, y=760.0) -> (0:w431:bool)
            n154 = case shown="True" w431 {
              tunnel: [w438 767] -> w435
              tunnel: w434 -> [_ _]
              tunnel: w432 -> [w440 _]
              tunnel: w430 -> [w436 _]
              frame False {
                n155 = Greater?(x=w440, y=760.0) -> (0:w437:bool)
                n156 = case shown="True" w437 {
                  tunnel: [w441 767] -> w438
                  tunnel: w436 -> [w441 _]
                  frame False {
                  }
                  frame True {
                  }
                }
              }
              frame True {
              }
            }
          }
        }
      }
    }
    n157 = feedback-in #10(w112) -> ()
    n158 = feedback #11(0.0) -> (w134:dbl)
    n159 = case shown="True" "Fly presence? J8" {
      tunnel: w138 -> [_ w343]
      tunnel: [0 w342] -> w127
      tunnel: w138 -> [_ w336]
      tunnel: w138 -> [_ w335]
      tunnel: w134 -> [_ w334]
      tunnel: w134 -> [_ w333]
      frame False {
      }
      frame True {
        n160 = Less?(x=w336, y=10.0) -> (x < y?=w339:bool)
        n161 = Greater?(x=w336, y=760.0) -> (0:w337:bool)
        n162 = Or(x=w337, y=w339) -> (x .or. y?=w341:bool)
        n163 = case shown="True" w341 {
          tunnel: w343 -> [w344 w350]
          tunnel: [w344 w351] -> w342
          tunnel: w335 -> [_ w345]
          tunnel: w334 -> [_ w348]
          tunnel: w333 -> [_ w346]
          frame False {
          }
          frame True {
            n164 = Greater?(x=w345, y=760.0) -> (0:w347:bool)
            n165 = case shown="False" w347 {
              tunnel: [w354 767] -> w351
              tunnel: w350 -> [_ _]
              tunnel: w348 -> [w356 _]
              tunnel: w346 -> [w352 _]
              frame False {
                n166 = Greater?(x=w356, y=760.0) -> (0:w353:bool)
                n167 = case shown="True" w353 {
                  tunnel: [w357 767] -> w354
                  tunnel: w352 -> [w357 _]
                  frame False {
                  }
                  frame True {
                  }
                }
              }
              frame True {
              }
            }
          }
        }
      }
    }
    n168 = feedback-in #11(w127) -> ()
    n169 = feedback #12(0.0) -> (w148:dbl)
    n170 = case shown="True" "Fly presence? J5" {
      tunnel: w151 -> [_ w371]
      tunnel: [0 w370] -> w128
      tunnel: w151 -> [_ w364]
      tunnel: w151 -> [_ w363]
      tunnel: w148 -> [_ w362]
      tunnel: w148 -> [_ w361]
      frame False {
      }
      frame True {
        n171 = Less?(x=w364, y=10.0) -> (x < y?=w367:bool)
        n172 = Greater?(x=w364, y=760.0) -> (0:w365:bool)
        n173 = Or(x=w365, y=w367) -> (x .or. y?=w369:bool)
        n174 = case shown="True" w369 {
          tunnel: w371 -> [w372 w378]
          tunnel: [w372 w379] -> w370
          tunnel: w363 -> [_ w373]
          tunnel: w362 -> [_ w376]
          tunnel: w361 -> [_ w374]
          frame False {
          }
          frame True {
            n175 = Greater?(x=w373, y=760.0) -> (0:w375:bool)
            n176 = case shown="False" w375 {
              tunnel: [w382 767] -> w379
              tunnel: w378 -> [_ _]
              tunnel: w376 -> [w384 _]
              tunnel: w374 -> [w380 _]
              frame False {
                n177 = Greater?(x=w384, y=760.0) -> (0:w381:bool)
                n178 = case shown="True" w381 {
                  tunnel: [w385 767] -> w382
                  tunnel: w380 -> [w385 _]
                  frame False {
                  }
                  frame True {
                  }
                }
              }
              frame True {
              }
            }
          }
        }
      }
    }
    n179 = feedback-in #12(w128) -> ()
    n180 = feedback #13(0.0) -> (w163:dbl)
    n181 = case shown="True" "Fly presence? J4" {
      tunnel: w166 -> [_ w399]
      tunnel: [0 w398] -> w129
      tunnel: w166 -> [_ w392]
      tunnel: w166 -> [_ w391]
      tunnel: w163 -> [_ w390]
      tunnel: w163 -> [_ w389]
      frame False {
      }
      frame True {
        n182 = Less?(x=w392, y=10.0) -> (x < y?=w395:bool)
        n183 = Greater?(x=w392, y=760.0) -> (0:w393:bool)
        n184 = Or(x=w393, y=w395) -> (x .or. y?=w397:bool)
        n185 = case shown="True" w397 {
          tunnel: w399 -> [w400 w406]
          tunnel: [w400 w407] -> w398
          tunnel: w391 -> [_ w401]
          tunnel: w390 -> [_ w404]
          tunnel: w389 -> [_ w402]
          frame False {
          }
          frame True {
            n186 = Greater?(x=w401, y=760.0) -> (0:w403:bool)
            n187 = case shown="False" w403 {
              tunnel: [w410 767] -> w407
              tunnel: w406 -> [_ _]
              tunnel: w404 -> [w412 _]
              tunnel: w402 -> [w408 _]
              frame False {
                n188 = Greater?(x=w412, y=760.0) -> (0:w409:bool)
                n189 = case shown="True" w409 {
                  tunnel: [w413 767] -> w410
                  tunnel: w408 -> [w413 _]
                  frame False {
                  }
                  frame True {
                  }
                }
              }
              frame True {
              }
            }
          }
        }
      }
    }
    n190 = feedback-in #13(w129) -> ()
    n191 = case shown="0, Default" "Choose which setup to look at" {
      tunnel: w133 -> [_ w319 w323 w327 w331]
      tunnel: [w313 w318 w322 w326 w330] -> w131
      tunnel: w112 -> [_ w317 _ _ _]
      tunnel: [w314 w317 w321 w325 w329] -> w130
      tunnel: w129 -> [_ _ w321 _ _]
      tunnel: w128 -> [_ _ _ w325 _]
      tunnel: w127 -> [_ _ _ _ w329]
      tunnel: [w313 w316 w320 w324 w328] -> w126
      tunnel: w125 -> [_ w316 _ _ _]
      tunnel: w124 -> [_ _ w320 _ _]
      tunnel: w123 -> [_ _ _ w324 _]
      tunnel: w122 -> [_ _ _ _ w328]
      frame 0, Default {
        w314 = 0.0 ("element")
        n192 = Initialize Array(w314, 768 ("dimension size")) -> (w313:dbl[])
      }
      frame 1 {
        n193 = Decimate 1D Array(w319) -> (w318:u16[])  [unwired: 3 out]
      }
      frame 2 {
        n194 = Decimate 1D Array(w323) -> (w322:u16[])  [unwired: 3 out]
      }
      frame 3 {
        n195 = Decimate 1D Array(w327) -> (w326:u16[])  [unwired: 3 out]
      }
      frame 4 {
        n196 = Decimate 1D Array(w331) -> (w330:u16[])  [unwired: 3 out]
      }
    }
    "Display Raw Data" <- w131
    "Fly real-time location" <- w130
    "Noise check" <- w126
    n197 = Subtract(x=w127, y=w134) -> (x-y=w135:dbl)
    n198 = Subtract(x=w112, y=w162) -> (x-y=w177:dbl)
    n199 = Subtract(x=w129, y=w163) -> (x-y=w164:dbl)
    n200 = Subtract(x=w128, y=w148) -> (x-y=w149:dbl)
    n201 = Build Array(w127, w91) -> (w108:dbl[])
    n202 = Build Array(w112, w93) -> (w105:dbl[])
    n203 = Build Array(w129, w94) -> (w111:dbl[])
    n204 = Build Array(w128, w92) -> (w109:dbl[])
    n205 = Absolute Value(x=w135) -> ()  [unwired: 1 out]
    n206 = Absolute Value(x=w177) -> ()  [unwired: 1 out]
    n207 = Absolute Value(x=w164) -> ()  [unwired: 1 out]
    n208 = Absolute Value(x=w149) -> ()  [unwired: 1 out]
    n209 = Enqueue Element(queue=w106, element=w108) -> ()  [unwired: 2 in, 3 out]
    n210 = Enqueue Element(queue=w104, element=w105) -> ()  [unwired: 2 in, 3 out]
    n211 = Enqueue Element(queue=w110, element=w111) -> ()  [unwired: 2 in, 3 out]
    n212 = Enqueue Element(queue=w107, element=w109) -> ()  [unwired: 2 in, 3 out]
    n213 = node-c288() -> ()  [unwired: 1 in, 1 out]
    "Host VI loop count" <- w121
  }
  n214 = timed-loop {
    tunnel: w2 -> [w507]
    tunnel: [w506] -> w86
    timing: w85 -> [_]
    timing-out: [_] -> w84
    i -> [w484]
    stop <- "Producer Loop Stop-2" stop-if-true
    n215 = node-c288() -> ()  [unwired: 1 in, 1 out]
    n216 = Subtract(x=4000.0, y="LED intensity J1") -> (x-y=w503:dbl)
    n217 = Subtract(x=4000.0, y="LED intensity J4") -> (x-y=w500:dbl)
    n218 = Subtract(x=4000.0, y="LED intensity J5") -> (x-y=w497:dbl)
    n219 = Subtract(x=4000.0, y="LED intensity J8") -> (x-y=w495:dbl)
    n220 = xnode "Read/Write Control"("FPGA VI Reference In"=w507, "LED intensity J1"="LED intensity J1", "Low Period (ticks) J1"=w503, "LED switch-1 J1"="LED switch-1 J1", "LED switch-2 J1"="LED switch-2 J1", "LED intensity J4"="LED intensity J4", "Low Period (ticks) J4"=w500, "LED switch-1 J4"="LED switch-1 J4", "LED switch-2 J4"="LED switch-2 J4", "LED intensity J5"="LED intensity J5", "Low Period (ticks) J5"=w497, "LED switch-1 J5"="LED switch-1 J5", "LED switch-2 J5"="LED switch-2 J5", "LED intensity J8"="LED intensity J8", "Low Period (ticks) J8"=w495, "LED switch-1 J8"="LED switch-1 J8", "LED switch-2 J8"="LED switch-2 J8") -> ("FPGA VI Reference Out"=w506:refnum<k20>)  [unwired: 1 in, 1 out]
    n221 = node-c288() -> ()  [unwired: 1 in, 1 out]
    "Loop count of LED" <- w484
  }
  n222 = while {
    tunnel: [w538] -> w21
    tunnel: w17 -> [w537]
    tunnel: w14 -> [w536]
    tunnel: [w535] -> w20
    tunnel: [w533] -> w19
    tunnel: [w532] -> w18
    tunnel: w15 -> [w531]
    tunnel: w16 -> [w530]
    tunnel: w4 -> [_]
    tunnel: w12 -> [w528]
    tunnel: [w527] -> w11
    tunnel: [w526] -> w10
    tunnel: [w525] -> w9
    tunnel: w7 -> [w524]
    tunnel: w6 -> [w523]
    tunnel: [w519] -> w5
    tunnel: w4 -> [w518]
    shift-right: [w512] -> _
    shift-left: w3 -> [w513]
    stop <- "Consumer Loop Stop" stop-if-true
    w529 = string[] ["Fly_position", "Laser_status"] ("channel name(s) in (Untitled)")
    w534 = "Measured Data" ("group name")
    n223 = Tick Count (ms)() -> (millisecond timer value=w512:u32)
    n224 = Subtract(x=w512, y=w513) -> (x-y=→"Consumer Loop Time":u32)
    n225 = Dequeue Element(queue=w518) -> (queue out=w519:refnum<queue>, element=w510:dbl[])  [unwired: 2 in, 2 out]
    n226 = Dequeue Element(queue=w528) -> (queue out=w527:refnum<queue>, element=w517:dbl[])  [unwired: 2 in, 2 out]
    n227 = Dequeue Element(queue=w524) -> (queue out=w526:refnum<queue>, element=w521:dbl[])  [unwired: 2 in, 2 out]
    n228 = Dequeue Element(queue=w523) -> (queue out=w525:refnum<queue>, element=w515:dbl[])  [unwired: 2 in, 2 out]
    n229 = call-poly <vilib>:"Array To Matrix.vi"("Real 1D Array"=w515) -> ("Real Matrix (Column Vector)"=w514:T5)
    n230 = call-poly <vilib>:"Array To Matrix.vi"("Real 1D Array"=w517) -> ("Real Matrix (Column Vector)"=w516:T5)
    n231 = call-poly <vilib>:"Array To Matrix.vi"("Real 1D Array"=w521) -> ("Real Matrix (Column Vector)"=w520:T5)
    n232 = call-poly <vilib>:"Array To Matrix.vi"("Real 1D Array"=w510) -> ("Real Matrix (Column Vector)"=w522:T5)
    n233 = TDMS Write(0:w537, 5:w534, 7:w529, 9:w522) -> (4:w538:refnum<k34>)  [unwired: 2 in, 3 out]
    n234 = TDMS Write(0:w531, 5:w534, 7:w529, 9:w520) -> (4:w533:refnum<k34>)  [unwired: 2 in, 3 out]
    n235 = TDMS Write(0:w536, 5:w534, 7:w529, 9:w516) -> (4:w535:refnum<k34>)  [unwired: 2 in, 3 out]
    n236 = TDMS Write(0:w530, 5:w534, 7:w529, 9:w514) -> (4:w532:refnum<k34>)  [unwired: 2 in, 3 out]
  }
  n237 = TDMS Close(11:w19) -> ()  [unwired: 1 in, 2 out]
  n238 = TDMS Close(11:w21) -> ()  [unwired: 1 in, 2 out]
  n239 = TDMS Close(11:w20) -> ()  [unwired: 1 in, 2 out]
  n240 = TDMS Close(11:w18) -> ()  [unwired: 1 in, 2 out]
  n241 = Release Queue(queue=w5) -> ()  [unwired: 2 in, 3 out]
  n242 = Release Queue(queue=w11) -> ()  [unwired: 2 in, 3 out]
  n243 = Release Queue(queue=w10) -> ()  [unwired: 2 in, 3 out]
  n244 = Release Queue(queue=w9) -> ()  [unwired: 2 in, 3 out]
  n245 = node-c288(w84) -> ()  [unwired: 1 out]
  n246 = xnode "Close FPGA VI Reference"("FPGA VI Reference In"=w86) -> ()  [unwired: 1 in, 1 out]
  n247 = node-c288(w89) -> ()  [unwired: 1 out]
  n248 = disable-structure shown="Disabled" {
    frame Disabled {
      n249 = TDMS Close() -> ()  [unwired: 2 in, 2 out]
      n250 = TDMS Close() -> ()  [unwired: 2 in, 2 out]
      n251 = TDMS Close() -> ()  [unwired: 2 in, 2 out]
      n252 = TDMS Close() -> ()  [unwired: 2 in, 2 out]
    }
    frame Enabled {
    }
  }
  n253 = xnode "Close FPGA VI Reference"("FPGA VI Reference In"=w1) -> ()  [unwired: 1 in, 1 out]
  n254 = xnode "Close FPGA VI Reference"("FPGA VI Reference In"=w87) -> ()  [unwired: 1 in, 1 out]
